vi "ReadTilesheetFromPNG.vi"(8 "error in (no error)":errorcluster, 11 "path to PNG file":path=path "/home/lvuser/natinst/bin/data/Aesomatica_16x16.png") -> (0 "error out":errorcluster, 3 "TileBufferData":fxp<+,3,3>[](array[numeric]))   [LabVIEW 2019, in "RT_Game.lvlib" / "Engine.lvclass"]
uses:
  Engine.lvclass
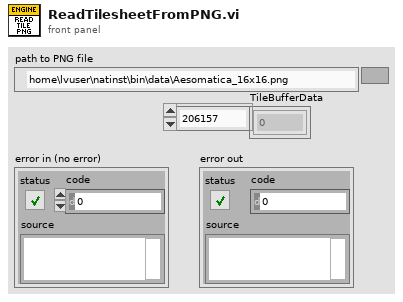
[diagram p1: front panel]
types:
  T1 = typedef "Color (U64)" = cluster{"Plane 3 (Blue)":u16, "Plane 2 (Green)":u16, "Plane 1 (Red)":u16, "Plane 4 (alpha)":u16}
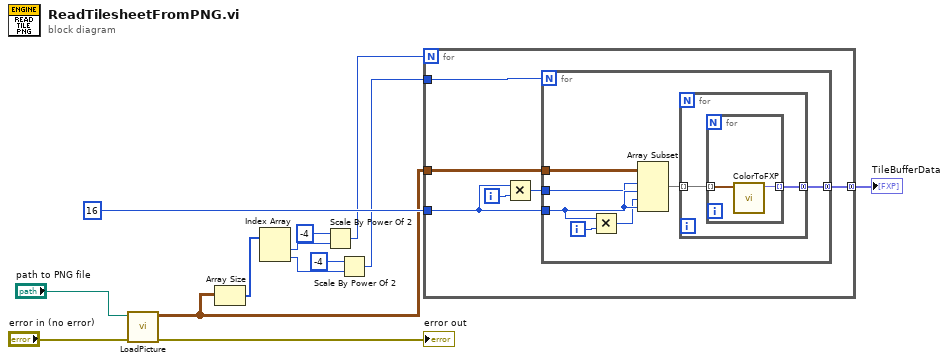
[diagram p0: block diagram]
diagram:
  n1 = call "LoadPicture.vi"("error in (no error)"="error in (no error)", "path to PNG file"="path to PNG file") -> ("error out"=→"error out":errorcluster, "Image Pixels (U64)"=w8:T1[][])  [unwired: 8 in]
  n2 = Array Size(array=w8) -> (size(s)=w7:i32[])
  n3 = Index Array(array=w7) -> (element #1=w6:i32, element #2=w2:i32)  [unwired: 2 in]
  n4 = Scale By Power Of 2(n=i16 -4, x=w6) -> (x*2^n=w4:i32)
  n5 = Scale By Power Of 2(n=i16 -4, x=w2) -> (x*2^n=w1:i32)
  n6 = for {
    N: w4 -> [_]
    tunnel: w8 -> [w19]
    tunnel: 16 ("length") -> [w16]
    tunnel: [w18] -> w12 mode=concatenating
    tunnel: w1 -> [w14]
    i -> [w17]
    n7 = Multiply(x=w16, y=w17) -> (x*y=w15:i32)
    n8 = for {
      N: w14 -> [_]
      tunnel: w19 -> [w26]
      tunnel: w16 -> [w24]
      tunnel: [w23] -> w18 mode=concatenating
      tunnel: w15 -> [w20]
      i -> [w25]
      n9 = Multiply(x=w24, y=w25) -> (x*y=w21:i32)
      n10 = Array Subset(array=w26, index (row)=w20, length (row)=w24, index (col)=w21, length (col)=w24) -> (w22:T1[][])
      n11 = for {
        tunnel: w22 -> [w28] mode=indexing
        tunnel: [w27] -> w23 mode=concatenating
        n12 = for {
          tunnel: w28 -> [w30] mode=indexing
          tunnel: [w29] -> w27 mode=indexing
          n13 = call "ColorToFXP.vi"("Color (U64)"=w30) -> ("Numeric"=w29:fxp<+,3,3>)  [unwired: 10 in]
        }
      }
    }
  }
  "TileBufferData" <- w12
